vi "FindWindowEx.vi"(8 "error in (no error)":errorcluster, 9 "window name (\"\")":string, 10 "hWndChildAfter\n(NULL)":T1, 11 "hWndParent\n(NULL)":T1) -> (0 "error out":errorcluster, 3 "hWnd":T1)   [LabVIEW 2011]
doc: "FindWindowEx\nThe FindWindowEx function retrieves a handle to a window whose class name and window name match the specified strings. The function searches child windows, beginning with the one following the given child window. This function does not perform a case-sensitive search. \n\nHWND FindWindowEx(\n HWND hwndParent, // handle to parent window\n HWND hwndChildAfter, // handle to a child window\n LPCTSTR lpszClass, // pointer to class name\n LPCTSTR lpszWindow // pointer to window name\n);\n \nParameters\nhwndParent \nHandle to the parent window whose child windows are to be searched. \nIf hwndParent is NULL, the function uses the desktop window as the parent window. The function searches among windows that are child windows of the desktop. \n\nWindows NT 5.0 and later: If hwndParent is HWND_MESSAGE, the function searches all message-only windows. \n\nhwndChildAfter \nHandle to a child window. The search begins with the next child window in the Z order. The child window must be a direct child window of hwndParent, not just a descendant window. \nIf hwndChildAfter is NULL, the search begins with the first child window of hwndParent. \n\nNote that if both hwndParent and hwndChildAfter are NULL, the function searches all top-level and message-only windows. \n\nlpszClass \nPointer to a null-terminated string that specifies the class name or is an atom that identifies the class-name string. If this parameter is an atom, it must be a global atom created by a previous call to theGlobalAddAtom function. The atom, a 16-bit value, must be placed in the low-order word of lpszClass; the high-order word must be zero. \nlpszWindow \nPointer to a null-terminated string that specifies the window name (the window's title). If this parameter is NULL, all window names match. \nReturn Values\nIf the function succeeds, the return value is a handle to the window that has the specified class and window names.\n\nIf the function fails, the return value is NULL. To get extended error information, callGetLastError."
uses:
  hWnd.ctl
  user32.dll
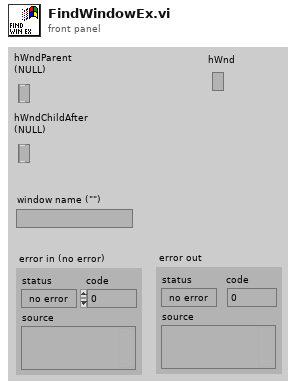
[diagram p1: front panel]
types:
  T1 = typedef "hWnd.ctl" = refnum<k1>
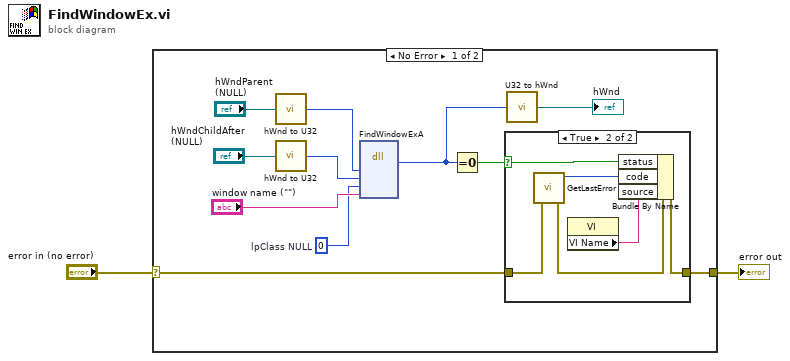
[diagram p0: block diagram]
diagram:
  n1 = case shown="No Error" "error in (no error)" {
    selector: "error in (no error)" -> [w8 w21]
    tunnel: [w12 w21] -> w2
    frame No Error {
      w3 = u32 0  # lpClass NULL
      n2 = call "hWnd to U32.vi"("hWnd"="hWndParent\n(NULL)") -> ("hWnd"=w6:u32)  [unwired: 4 out]
      n3 = call "hWnd to U32.vi"("hWnd"="hWndChildAfter\n(NULL)") -> ("hWnd"=w4:u32)  [unwired: 4 out]
      n4 = dll-call lib="User32.dll" fn="FindWindowExA" label="FindWindowEx"("hWndParent"=w6, "hWndChildAfter"=w4, "lpClass"=w3, "lpWindow"="window name (\"\")") -> ("hWnd"=w11:u32)  [unwired: 7 in, 2 out]
      n5 = Equal To 0?(x=w11) -> (x = 0?=w9:bool)
      n6 = case shown="True" w9 {
        selector: w9 -> [_ w19]
        tunnel: [w14 w20] -> w12
        tunnel: w8 -> [w14 w15]
        frame False {
        }
        frame True {
          n7 = call "GetLastError.vi"("error in (no error)"=w15) -> ("error out"=w17:errorcluster, "CODE"=w18:i32)  [unwired: 5 out]
          n8 = property class="VI"() -> ("VI Name"=w16:string)  [unwired: 2 in, 2 out]
          n9 = Bundle By Name(cluster=w17, "status"=w19, "code"=w18, "source"=w16) -> (w20:errorcluster)
        }
      }
      n10 = call "U32 to hWnd.vi"("hWnd"=w11) -> ("hWnd"=→"hWnd":T1)  [unwired: 4 out]
    }
    frame Error {
    }
  }
  "error out" <- w2
